vi "FGV_MIDAS_ODB_data.vi"(9 "input cluster":T1, 11 "Enum":T2) -> (1 "MIDAS_ODB_Entry":T1, 3 "Found Entry":bool)   [LabVIEW 2018, in "feGEM DataPacker.lvlib"]
uses:
  feGEM DataPacker.lvlib
  MIDAS_ODB_Set_Get_Clear_Enum.ctl
  DataStructures/MIDAS_ODB_Entry.ctl
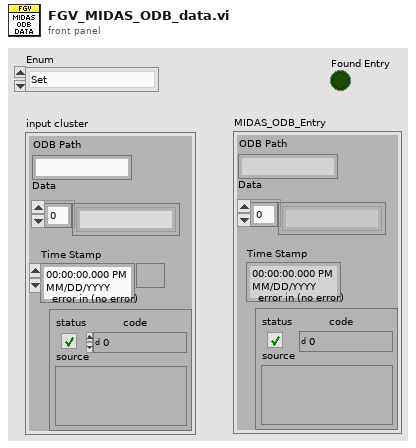
[diagram p1: front panel]
types:
  T1 = typedef "feGEM DataPacker.lvlib/MIDAS_ODB_Entry.ctl" = cluster{"ODB Path":string, "Data":string[], "Time Stamp":timestamp, "error in (no error)":errorcluster}
  T2 = typedef "feGEM DataPacker.lvlib/MIDAS_ODB_Set_Get_Clear_Enum.ctl" = enum16{"Set", "Get", "Clear"}
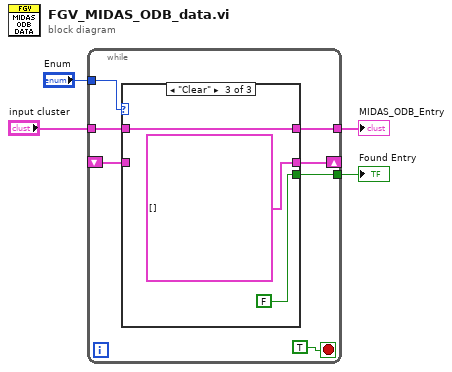
[diagram p0: block diagram]
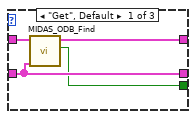
[diagram p2: hidden frame]
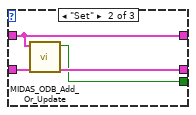
[diagram p3: hidden frame]
diagram:
  n1 = while {
    shift-right: [w10] -> _
    shift-left: _ -> [w11]
    tunnel: "input cluster" -> [w9]
    tunnel: "Enum" -> [w8]
    tunnel: [w6] -> w2
    tunnel: [w5] -> w1
    stop <- TRUE stop-if-true
    n2 = case shown="\"Clear\"" w8 {
      tunnel: [w14 w18 T1[] [] ("Output Array")] -> w10
      tunnel: w11 -> [w14 w19 _]
      tunnel: w9 -> [w15 w17 w22]
      tunnel: [w13 w17 w22] -> w6
      tunnel: [w12 w16 FALSE ("Entry Already Exists")] -> w5
      frame "Get", Default {
        n3 = call "MIDAS_ODB_Find.vi"("Array"=w14, "input cluster"=w15) -> ("Found Entry"=w12:bool, "MIDAS_ODB_Entry"=w13:T1)  [unwired: 8 in]
      }
      frame "Set" {
        n4 = call "MIDAS_ODB_Add_Or_Update.vi"("Input Array"=w19, "input cluster"=w17) -> ("Output Array"=w18:T1[], "Entry Already Exists"=w16:bool)  [unwired: 8 in]
      }
      frame "Clear" {
      }
    }
  }
  "MIDAS_ODB_Entry" <- w2
  "Found Entry" <- w1
